vi "Set message.vi"(10 "WampMessage MsgPack":refnum<class "WampMessage MsgPack.lvclass">, 11 "HandleGoodby MsgPack in":refnum<class "HandleGoodby MsgPack.lvclass">) -> (3 "HandleGoodby MsgPack out":refnum<class "HandleGoodby MsgPack.lvclass">)   [LabVIEW 2020, in "wamplv.lvlib" / "HandleGoodby MsgPack.lvclass"]
uses:
  HandleGoodby MsgPack.lvclass
  HandleGoodby MsgPack.lvclass/HandleGoodby MsgPack.ctl
  SerialisedMessages/MsgPackMessage/WampMessage MsgPack.lvclass
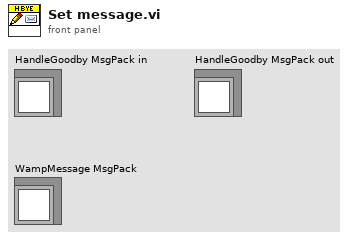
[diagram p1: front panel]
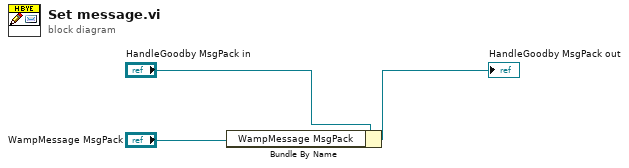
[diagram p0: block diagram]
diagram:
  n1 = Bundle By Name(cluster="HandleGoodby MsgPack in", "WampMessage MsgPack"="WampMessage MsgPack") -> (→"HandleGoodby MsgPack out":refnum<class "HandleGoodby MsgPack.lvclass">)
